vi "Get Inline Plugin.vi"(10 "index":i32, 11 "Framework in":refnum<class "Framework.lvclass">) -> (2 "Inline Plugin":refnum<class "Plugin.lvclass">, 3 "Framework out":refnum<class "Framework.lvclass">)   [LabVIEW 2017, in "DSF Core.lvlib" / "Framework.lvclass"]
uses:
  Framework.lvclass
  Plugin/Plugin.lvclass
  Framework.lvclass/Framework.ctl
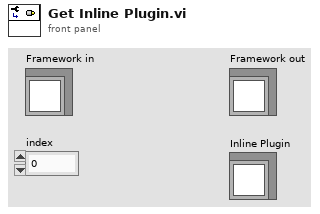
[diagram p1: front panel]
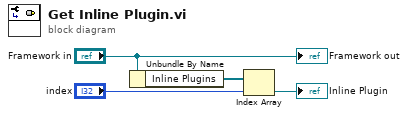
[diagram p0: block diagram]
diagram:
  n1 = Unbundle By Name("Framework in") -> ("Inline Plugins"=w1:refnum<class "Plugin.lvclass">[])
  n2 = Index Array(array=w1, index="index") -> (element=→"Inline Plugin":refnum<class "Plugin.lvclass">)
  "Framework out" <- "Framework in"
